vi "ex9-3.vi"() -> ()   [LabVIEW 2013]
uses:
  <vilib>/NXT/NXT Controls/ConnectionType.ctl
  <vilib>/NXT/Dual Mode Library/Sensors/EV3_Color_Reflect.vi
  <vilib>/NXT/Dual Mode Library/Sensors/EV3_Gyro_Angle.vi
panel:
  out "#2 - EV3 Color":sgl(graph)
  out "#1 - EV3 Gyro":sgl(graph)
  in  "Motor Power":dbl(slide) scale=-100.0..100.0
  in  "Steering":dbl(knob) scale=-100.0..100.0
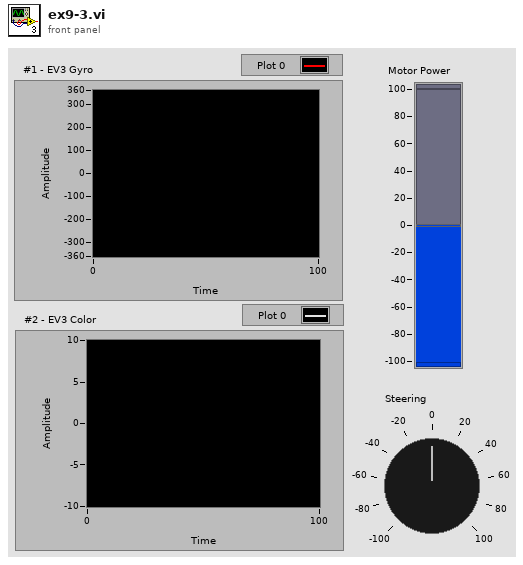
[diagram p1: front panel]
types:
  T1 = typedef "ConnectionType.ctl" = enum16{"Bluetooth", "USB", "WiFi"}
  T2 = typedef "LVHSConnector.ctl" = refnum<class "BrickReference.lvclass">
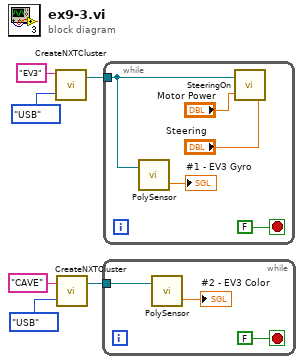
[diagram p0: block diagram]
diagram:
  n1 = call <vilib>:"CreateNXTCluster.vi"("Connection Type"=ConnectionType."USB", "NXT/EV3 name"="EV3") -> ("NXT/EV3"=w4:T2)  [unwired: 2 in]
  n2 = call <vilib>:"CreateNXTCluster.vi"("Connection Type"=ConnectionType."USB", "NXT/EV3 name"="CAVE") -> ("NXT/EV3"=w1:T2)  [unwired: 2 in]
  n3 = while {
    tunnel: w1 -> [w9]
    stop <- FALSE stop-if-true
    n4 = call-poly <vilib>:"PolySensor.vi"("NXT/EV3"=w9) -> ("Scaled Value"=→"#2 - EV3 Color":sgl)  [unwired: 2 in, 1 out]
  }
  n5 = while {
    tunnel: w4 -> [w14]
    stop <- FALSE stop-if-true
    n6 = call-poly <vilib>:"PolySensor.vi"("NXT/EV3"=w14) -> ("Degrees"=→"#1 - EV3 Gyro":sgl)  [unwired: 2 in, 1 out]
    n7 = call <vilib>:"SteeringOn.vi"("Power (75)"="Motor Power", "Steering (100)"="Steering", "NXT/EV3"=w14) -> ()  [unwired: 1 in, 1 out]
  }
